vi "TestPublishRate.vi"(8 "error in (no error)":errorcluster, 11 "TestPublishRate In":refnum<class "TestPublishRate.lvclass">) -> (0 "error out":errorcluster, 3 "TestPublishRate Out":refnum<class "TestPublishRate.lvclass">)   [LabVIEW 2015, in "TestPublishRate.lvclass"]
uses:
  TestPublishRate.lvclass
  Framework/IViewModel/IViewModel/IViewModel.lvclass
  Framework/IViewable/IViewable/IViewable.lvclass
  Doubles/TestModelFastPublish/TestModelFastPublish.lvclass
  Framework/Mediator/Mediator/Mediator.lvclass
  Framework/SubscriptionPolicy/ValueChangeSubscription/ValueChangeSubscription.lvclass/ValueChangeSubscription.ctl
  Framework/IViewModel/IViewModel/IViewModel.lvclass/IViewModel.ctl
  Framework/IViewManager/IViewManager Messages/Launch Nested Views Msg/Launch Nested Views Msg.lvclass/Launch Nested Views Msg.ctl
  Framework/IViewManager/IViewManager/IViewManager.lvclass/IViewManager.ctl
  Framework/IObserver/IObserver Messages/Subscribe Msg/Subscribe Msg.lvclass/Subscribe Msg.ctl
  <vilib>/ActorFramework/Message Enqueuer/Message Enqueuer.lvclass/Message Enqueuer.ctl
  <vilib>/ActorFramework/Stop Msg/Stop Msg.lvclass/Stop Msg.ctl
  <vilib>/Analysis/baseanly.llb/Mean (DBL).vi
  Framework/IViewManager/IViewManager Messages/Launch Nested Views Msg/Build Launch Nested Views Msg.vi
  Framework/IViewManager/IViewManager/Write Startup Launch Nested Views Msg.vi
  <vilib>/ActorFramework/Message Enqueuer/Enqueue.vi
  <vilib>/ActorFramework/Message Enqueuer/Enqueue Critical.vi
  <vilib>/ActorFramework/Message Priority Queue/Priority Enqueue.vi
  Framework/IViewManager/IViewManager Messages/Launch Nested Views Msg/Launch Nested Views Msg.lvclass
  Framework/SubscriptionPolicy/ValueChangeSubscription/ValueChangeSubscription.lvclass
  Framework/IObserver/IObserver Messages/Subscribe Msg/Subscribe Msg.lvclass
  <vilib>/ActorFramework/Stop Msg/Stop Msg.lvclass
  Framework/Transport/QueueTransport/QueueTransport.lvclass
  <vilib>/ActorFramework/Actor/Actor.lvclass
  Framework/IMediator/SubscriptionRequest/SubscriptionRequest.lvclass
  Framework/IMediator/ISubscriptionPolicy/ISubscriptionPolicy.lvclass
  <vilib>/Analysis/NI_AALBase.lvlib
panel:
  out "Iteration":i32
  out "Transmission Times":dbl[](graph)
  out "Actual Publish Period":dbl[](graph)
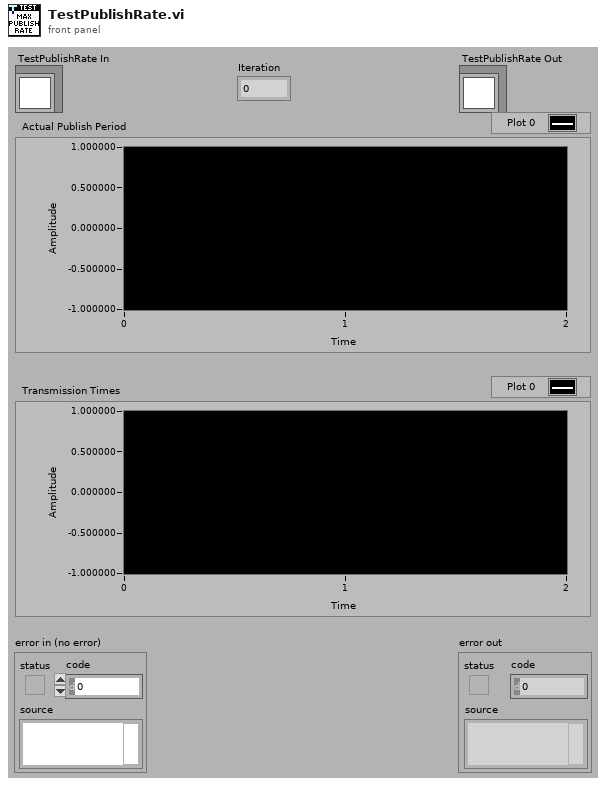
[diagram p1: front panel]
types:
  T1 = cluster{"Data":variant, "Publication Time":timestamp}
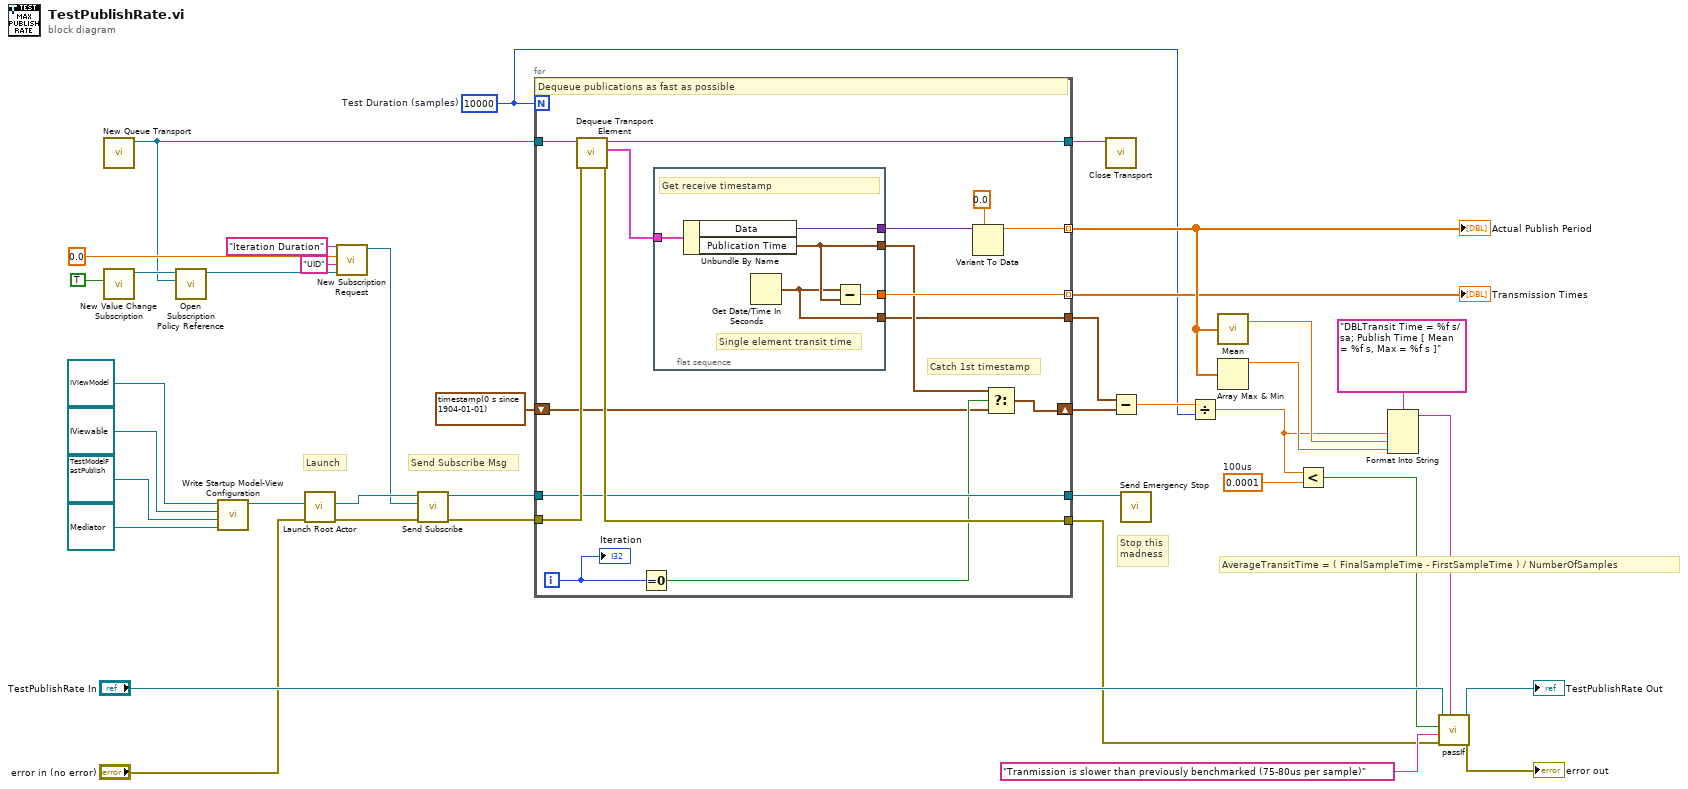
[diagram p0: block diagram]
diagram:
  w6 = 0.0001  # 100us
  w2 = 10000  # Test Duration (samples)
  # "AverageTransitTime = ( FinalSampleTime - FirstSampleTime ) / NumberOfSamples"
  # "Stop this\nmadness"
  # "Send Subscribe Msg"
  # "Launch"
  n1 = call "New Queue Transport.vi"() -> ("QueueTransport Out"=w1:refnum<class "QueueTransport.lvclass">)  [unwired: 10 in, 1 out]
  n2 = call "New Value Change Subscription.vi"("Ignore Past Updates? (F)"=TRUE) -> ("ValueChangeSubscription Out"=w29:refnum<class "ValueChangeSubscription.lvclass">)  [unwired: 10 in]
  n3 = call "Open Subscription Policy Reference.vi"("Transport"=w1, "SubscriptionPolicy"=w29) -> ("Subscription Policy"=w28:refnum<data-value>)  [unwired: 8 in, 1 out]
  n4 = call "Write Startup Model-View Configuration.vi"("Mediator"=refnum<class "Mediator.lvclass"> refnum, "Model"=refnum<class "TestModelFastPublish.lvclass"> refnum, "Startup View Configuration"=refnum<class "IViewable.lvclass"> refnum, "IViewModel In"=refnum<class "IViewModel.lvclass"> refnum) -> ("IViewModel Out"=w31:refnum<class "IViewModel.lvclass">)  [unwired: 7 in]
  n5 = call <vilib>:"Launch Root Actor.vi"("error in (no error)"="error in (no error)", "Actor"=w31) -> ("error out"=w23:errorcluster, "Actor's Enqueuer"=w30:refnum<class "Message Enqueuer.lvclass">)  [unwired: 8 in]
  n6 = call "New Subscription Request.vi"("Subscription Policy"=w28, "Unique Subscriber ID"="UID", "Type"=0.0, "Topic Name"="Iteration Duration") -> ("SubscriptionRequest"=w25:refnum<class "SubscriptionRequest.lvclass">)  [unwired: 7 in]
  n7 = call "Send Subscribe.vi"("error in (no error)"=w23, "SubscriptionRequest"=w25, "Message Enqueuer"=w30) -> ("error out"=w22:errorcluster, "Message Enqueuer out"=w24:refnum<class "Message Enqueuer.lvclass">)  [unwired: 7 in]
  n8 = for {
    N: w2 -> [_]
    tunnel: w24 -> [w48]
    tunnel: w22 -> [w52]
    tunnel: w1 -> [w53]
    tunnel: [w50] -> w16 mode=indexing
    tunnel: [w49] -> w13 mode=indexing
    tunnel: [w51] -> w3
    tunnel: [w48] -> w15
    tunnel: [w47] -> w14
    shift-right: [w46] -> w10
    shift-left: timestamp(0 s since 1904-01-01) ("Publication Time") -> [w42]
    tunnel: [w41] -> w11
    i -> [w44]
    # "Catch 1st timestamp"
    # "Dequeue publications as fast as possible"
    n9 = call "Dequeue Transport Element.vi"("error in (no error)"=w52, "QueueTransport in"=w53) -> ("error out"=w51:errorcluster, "Element"=w55:T1, "QueueTransport out"=w47:refnum<class "QueueTransport.lvclass">)  [unwired: 6 in, 1 out]
    n10 = Equal To 0?(x=w44) -> (x = 0?=w43:bool)
    n11 = flat-sequence {
      tunnel: w55 -> [w60]
      tunnel: [w59] -> w54
      tunnel: [w58] -> w49
      tunnel: [w57] -> w45
      tunnel: [w56] -> w41
      frame #0 {
        # "Single element transit time"
        # "Get receive timestamp"
        n12 = Unbundle By Name(w60) -> ("Data"=w59:variant, "Publication Time"=w57:timestamp)
        n13 = Get Date/Time In Seconds() -> (seconds since 1Jan1904=w56:timestamp)
        n14 = Subtract(x=w56, y=w57) -> (x-y=w58:dbl)
      }
    }
    n15 = Variant To Data(type=0.0, Variant=w54) -> (data=w50:dbl)  [unwired: 1 in, 1 out]
    n16 = Select(t=w45, s=w43, f=w42) -> (s? t:f=w46:timestamp)
    "Iteration" <- w44
  }
  "Actual Publish Period" <- w16
  "Transmission Times" <- w13
  n17 = call-dynamic "Close Transport.vi"("QueueTransport in"=w14) -> ()  [unwired: 10 in, 1 out]
  n18 = Subtract(x=w11, y=w10) -> (x-y=w9:dbl)
  n19 = call <vilib>:"Send Emergency Stop.vi"("Message Enqueuer"=w15) -> ()  [unwired: 10 in, 1 out]
  n20 = Divide(x=w9, y=w2) -> (x/y=w7:dbl)
  n21 = call-poly <vilib>:"Mean.vi"("X"=w16) -> ("mean"=w18:dbl)  [unwired: 1 out]
  n22 = Array Max & Min(array=w16) -> (max value=w17:dbl)  [unwired: 3 out]
  n23 = Less?(x=w7, y=w6) -> (x < y?=w5:bool)
  n24 = Format Into String(format string="DBLTransit Time = %f s/sa; Publish Time [ Mean = %f s, Max = %f s ]", w7, w18, w17) -> (resulting string=w8:string)  [unwired: 2 in, 1 out]
  n25 = call-dynamic "passIf.vi"("custom report message (\"\")"=w8, "error in (no error)"=w3, "message (\"\")"="Tranmission is slower than previously benchmarked (75-80us per sample)" ("message (\"\")"), "pass"=w5, "TestCase in"="TestPublishRate In") -> ("error out"=→"error out":errorcluster, "TestCase out"=→"TestPublishRate Out":refnum<class "TestPublishRate.lvclass">)  [unwired: 5 in]
